vi "getAmplitude.vi"(8 "error in (no error)":errorcluster, 11 "Model in":refnum<class "Model.lvclass">) -> (0 "error out":errorcluster, 2 "Result":dbl, 3 "Model out":refnum<class "Model.lvclass">)   [LabVIEW 2015, in "Model.lvclass"]
uses:
  Model.lvclass
  Model.lvclass/Model.ctl
  <vilib>/express/express arith-compare/Formula/XNode/ExpressFormulaBlockNode.xnode
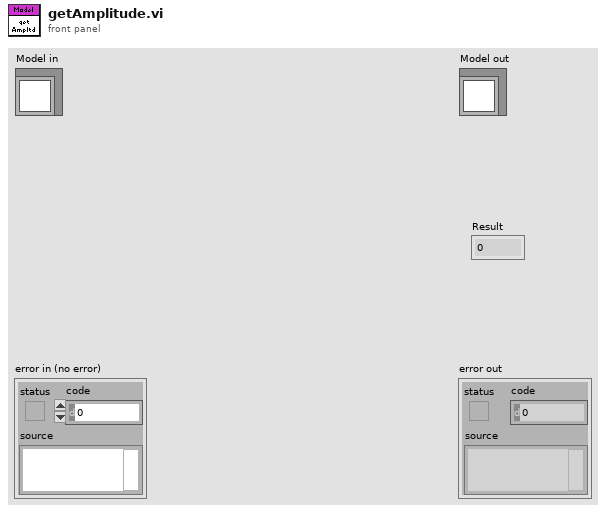
[diagram p1: front panel]
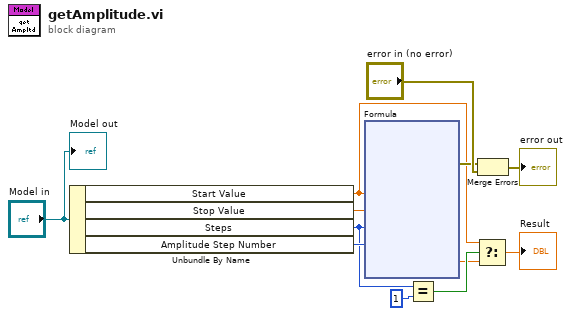
[diagram p0: block diagram]
diagram:
  n1 = Unbundle By Name("Model in") -> ("Start Value"=w1:dbl, "Stop Value"=w7:dbl, "Steps"=w6:u16, "Amplitude Step Number"=w8:u16)
  n2 = xnode "Formula"("START"=w1, "STOP"=w7, "STEPS"=w6, "STEP"=w8) -> ("Result"=w3:dbl, "error out"=w10:errorcluster)  [unwired: 1 in]
  n3 = Equal?(x=w6, y=u16 1) -> (x = y?=w4:bool)
  n4 = Select(t=w1, s=w4, f=w3) -> (s? t:f=→"Result":dbl)
  n5 = Merge Errors(w10, "error in (no error)") -> (→"error out":errorcluster)
  "Model out" <- "Model in"
